vi "Set LED Mode.vi"(0 "SerialPortRef 3":T1, 1 "Numeric":dbl, 11 "error in (no error)":errorcluster, 12 "Red":i32, 13 "Green":i32, 14 "Blue":i32) -> (4 "SerialPortRef":T1, 15 "error out":errorcluster)   [LabVIEW 2015]
uses:
  <vilib>/Rock Robotics/WPI/SerialPort/WPI_SerialPortRef.ctl
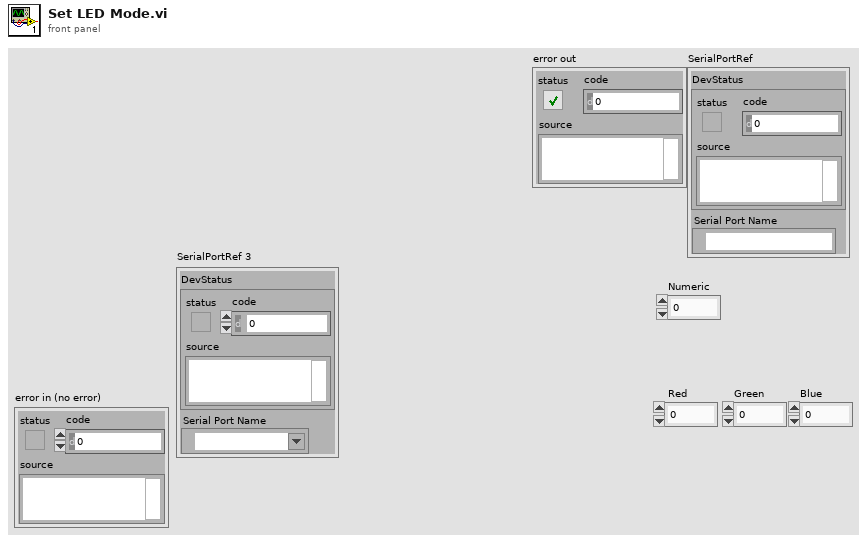
[diagram p1: front panel]
types:
  T1 = typedef "WPI_SerialPortRef.ctl" = cluster{"DevStatus":errorcluster, "Serial Port Name":refnum<visa-resource-name>}
  T2 = enum16{"Set Custom RGB", "Set Mode", "Set intensity"}
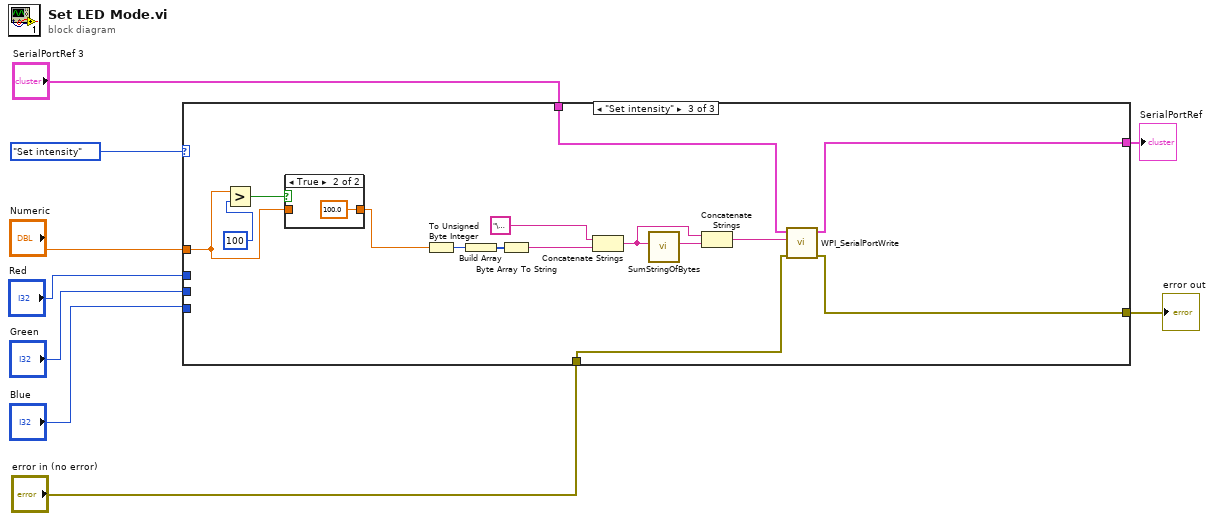
[diagram p0: block diagram]
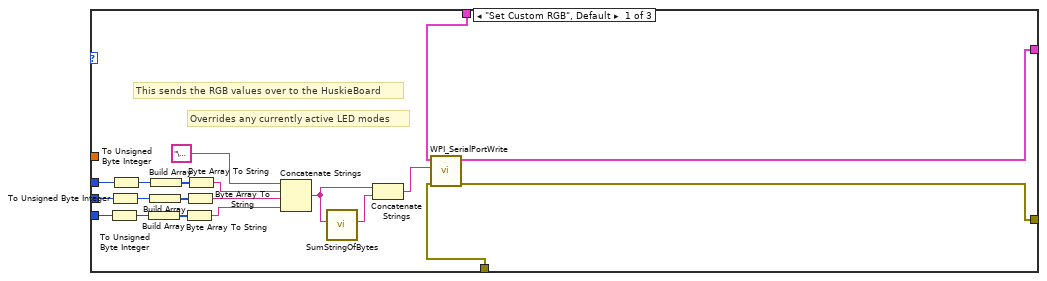
[diagram p2: hidden frame]
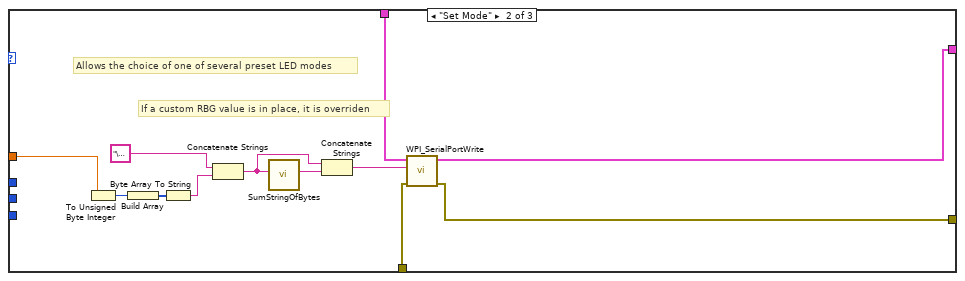
[diagram p3: hidden frame]
diagram:
  n1 = case shown="\"Set intensity\"" T2."Set intensity" ("Enum") {
    tunnel: "Numeric" -> [_ w39 w48]
    tunnel: "Red" -> [w27 _ _]
    tunnel: "Green" -> [w24 _ _]
    tunnel: "Blue" -> [w21 _ _]
    tunnel: "error in (no error)" -> [w13 w33 w44]
    tunnel: "SerialPortRef 3" -> [w12 w32 w45]
    tunnel: [w10 w30 w42] -> w3
    tunnel: [w11 w31 w43] -> w2
    frame "Set Custom RGB", Default {
      # "Overrides any currently active LED modes"
      # "This sends the RGB values over to the HuskieBoard"
      n2 = To Unsigned Byte Integer(number=w21) -> (unsigned 8bit integer=w23:u8)
      n3 = To Unsigned Byte Integer(number=w24) -> (unsigned 8bit integer=w26:u8)
      n4 = To Unsigned Byte Integer(number=w27) -> (unsigned 8bit integer=w29:u8)
      n5 = Build Array(w23) -> (w22:u8[])
      n6 = Build Array(w26) -> (w25:u8[])
      n7 = Build Array(w29) -> (w28:u8[])
      n8 = Byte Array To String(unsigned byte array=w22) -> (string=w20:string)
      n9 = Byte Array To String(unsigned byte array=w25) -> (string=w19:string)
      n10 = Byte Array To String(unsigned byte array=w28) -> (string=w18:string)
      n11 = Concatenate Strings("\u0015", w18, w19, w20) -> (w16:string)
      n12 = call "SumStringOfBytes.vi"("String Of Bytes"=w16) -> ("SumAsString"=w15:string)  [unwired: 10 in]
      n13 = Concatenate Strings(w16, w15) -> (w14:string)
      n14 = call <vilib>:"WPI_SerialPortWrite.vi"("error in (no error)"=w13, "Buffer"=w14, "SerialPortRef"=w12) -> ("error out"=w10:errorcluster, "SerialPortRef"=w11:T1)  [unwired: 6 in, 1 out]
    }
    frame "Set Mode" {
      # "If a custom RBG value is in place, it is overriden"
      # "Allows the choice of one of several preset LED modes"
      n15 = To Unsigned Byte Integer(number=w39) -> (unsigned 8bit integer=w41:u8)
      n16 = Build Array(w41) -> (w40:u8[])
      n17 = Byte Array To String(unsigned byte array=w40) -> (string=w38:string)
      n18 = Concatenate Strings("\u0014", w38) -> (w36:string)
      n19 = call "SumStringOfBytes.vi"("String Of Bytes"=w36) -> ("SumAsString"=w35:string)  [unwired: 10 in]
      n20 = Concatenate Strings(w36, w35) -> (w34:string)
      n21 = call <vilib>:"WPI_SerialPortWrite.vi"("error in (no error)"=w33, "Buffer"=w34, "SerialPortRef"=w32) -> ("error out"=w30:errorcluster, "SerialPortRef"=w31:T1)  [unwired: 6 in, 1 out]
    }
    frame "Set intensity" {
      n22 = Greater?(x=w48, y=100) -> (0:w50:bool)
      n23 = case shown="True" w50 {
        tunnel: w48 -> [w57 _]
        tunnel: [w57 100.0 ("Numeric")] -> w47
        frame False {
        }
        frame True {
        }
      }
      n24 = To Unsigned Byte Integer(number=w47) -> (unsigned 8bit integer=w56:u8)
      n25 = Build Array(w56) -> (w55:u8[])
      n26 = Byte Array To String(unsigned byte array=w55) -> (string=w46:string)
      n27 = Concatenate Strings("\u0016", w46) -> (w53:string)
      n28 = call "SumStringOfBytes.vi"("String Of Bytes"=w53) -> ("SumAsString"=w52:string)  [unwired: 10 in]
      n29 = Concatenate Strings(w53, w52) -> (w51:string)
      n30 = call <vilib>:"WPI_SerialPortWrite.vi"("error in (no error)"=w44, "Buffer"=w51, "SerialPortRef"=w45) -> ("error out"=w42:errorcluster, "SerialPortRef"=w43:T1)  [unwired: 6 in, 1 out]
    }
  }
  "error out" <- w3
  "SerialPortRef" <- w2
